vi "WPI_DigitalModuleSetPWM.vi"(6 "Indicate Zero":bool, 8 "error in (no error)":errorcluster, 9 "Speed":u16, 10 "PWMChannel":T1=enum."PWM 1") -> (0 "error out":errorcluster)   [LabVIEW 2017]
doc: "This software is licensed. Open the labview\\readme\\WPI Robotics Library Open Source License.txt file for more information."
uses:
  <vilib>/Rock Robotics/SystemInterfaces/DIO/FPGA_DIOPWMChannel.ctl
  <vilib>/Rock Robotics/SystemInterfaces/System/FPGA_SystemGet.vi
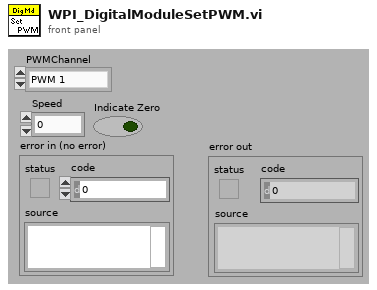
[diagram p1: front panel]
types:
  T1 = typedef "FPGA_DIOPWMChannel.ctl" = enum8{"PWM 0", "PWM 1", "PWM 2", "PWM 3", "PWM 4", "PWM 5", "PWM 6", "PWM 7", "PWM 8", "PWM 9", "PWM MXP 0", "PWM MXP 1", "PWM MXP 2", "PWM MXP 3", "PWM MXP 4", "PWM MXP 5", "PWM MXP 6", "PWM MXP 7", "PWM MXP 8", "PWM MXP 9", "Invalid"}
  T2 = typedef "FPGA_DIODevRef.ctl" = cluster{"DevStatus":errorcluster}
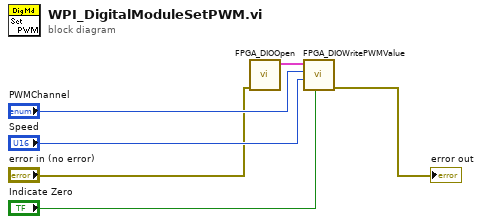
[diagram p0: block diagram]
diagram:
  n1 = call <vilib>:"FPGA_DIOOpen.vi"("error in (no error)"="error in (no error)") -> ("DIODeviceRef"=w3:T2)  [unwired: 1 in, 9 out]
  n2 = call <vilib>:"FPGA_DIOWritePWMValue.vi"("Indicate Zero"="Indicate Zero", "PWMValue"="Speed", "PWMChannel"="PWMChannel", "DIODeviceRef In"=w3) -> ("error out"=→"error out":errorcluster)  [unwired: 1 in, 6 out]
